vi "Create Controls in Configuration.vi"(8 "error in":errorcluster, 9 "vi refnum":refnum<vi>, 10 "control refnum in":refnum<vi>, 11 "cluster ref":refnum<vi>) -> (0 "error out":errorcluster, 3 "control refnum out":refnum<vi>)   [LabVIEW 2021, in "Converter.lvlib"]
uses:
  Converter.lvlib
  <vilib>/Utility/miscctls.llb/LVPositionTypeDef.ctl
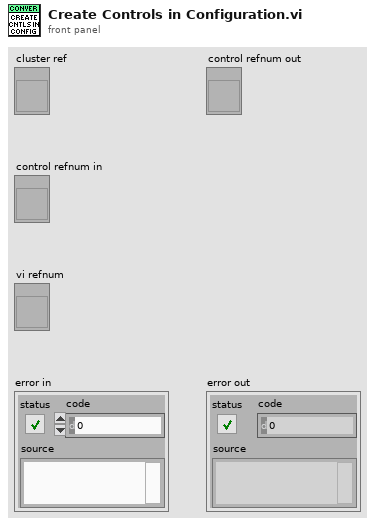
[diagram p1: front panel]
types:
  T1 = typedef "LVPositionTypeDef.ctl" = cluster{"Left":i32, "Top":i32}
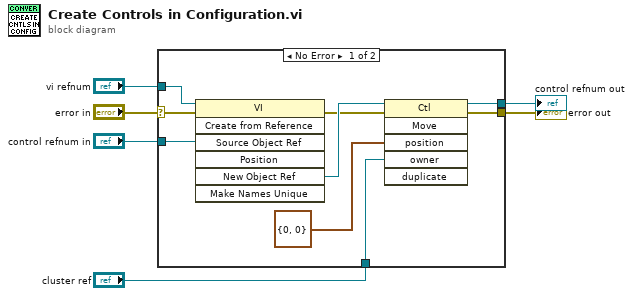
[diagram p0: block diagram]
diagram:
  n1 = case shown="No Error" "error in" {
    selector: "error in" -> [w12 w16]
    tunnel: [w8 _] -> w6
    tunnel: [w7 w16] -> w5
    tunnel: "control refnum in" -> [w15 _]
    tunnel: "cluster ref" -> [w14 _]
    tunnel: "vi refnum" -> [w13 _]
    frame No Error {
      n2 = invoke class="VI" method="Create from Reference"(reference=w13, error in=w12, "Source Object Ref"=w15) -> (error out=w9:errorcluster, "New Object Ref"=w10:refnum<vi>)  [unwired: 4 in, 5 out]
      n3 = invoke class="Ctl" method="Move"(reference=w10, error in=w9, "position"=T1 {"Left"=0, "Top"=0}, "owner"=w14) -> (reference out=w8:refnum<vi>, error out=w7:errorcluster)  [unwired: 2 in, 4 out]
    }
    frame Error {
    }
  }
  "control refnum out" <- w6
  "error out" <- w5
